vi "TLB Native Dynamic Events ver 0.08c.vi"() -> ()   [LabVIEW 2018]
uses:
  Labview Training Phase 2/Enum Controls/States for Action Engine.ctl
  Type def/TLB event states.ctl
  Type def/TLB MHL States.ctl
  <vilib>/Studica/Studica Toolkit/Background/I2C Channel.ctl
  <vilib>/myRIO/Common/Instrument Driver Framework/myRIO v1.0/AI/typedefs/AI Channels Enum.ctl
  <vilib>/myRIO/Common/Instrument Driver Framework/myRIO v1.0/AI/typedefs/AI Channels List.ctl
  Type def/Type def.ctl
  <vilib>/Studica/Studica Blackhawk/Blackhawk.lvlib
  <vilib>/Studica/Studica Toolkit/Background/Mxp Selection.ctl
  <vilib>/Studica/Studica Toolkit/Background/DIO Channel.ctl
  <vilib>/NI_Real-Time Target Support.lvlib
  <vilib>/ptbypt/NI_PtbyPt.lvlib
  <vilib>/addons/control/pid/NI_PID_pid.lvlib
  Underlying VI's/Webcam FGV Low level ver/State control.ctl
  <vilib>/userdefined/High Color/IMAQdx.ctl
  <vilib>/Studica/Studica Toolkit/NavX/NavX.lvlib
  <vilib>/addons/control/pid/pid.llb/PID (DBL).vi
panel:
  out "Displacement":T1
  out "Yaw":dbl
  out "Speed and distance cluster":T2
  out "Output":dbl
  in  "SENSOR":bool
  out "Decision":i8
  out "Manual Zero Yaw":bool
  in  "error in (no error)":errorcluster
  in  "RED LED State":enum16{"OFF", "ON", "BLINK"}(ring)
  in  "GREEN LED State":enum16{"OFF", "ON", "BLINK"}(ring)
  in  "Red LED":bool
  in  "Green LED":bool
  out "Input state":i8
  out "Waveform Chart 2":dbl(graph)
  out "Waveform Chart":dbl(graph)
  in  "STOP":bool
  out "DIO 0":bool
  out "DIO 1":bool
  out "Limit Switch Array":bool[](array[boolean])
  out "error out":errorcluster
  out "L/R average":fxp<+,64,64>
  out "Right Ultrasonic":fxp<+,64,16>
  out "Left Ultrasonic":fxp<+,64,16>
  out "Right IR Sensor":dbl
  out "Left IR Sensor":dbl
  out "Object detection count":T3
  out "Camera error":errorcluster
  in  "Servo Angle":u8(slide) scale=0.0..180.0
  in  "On/Off":bool
  out "Error":errorcluster
  out "element":T4
  out "Action Queue Items":i32
  out "State Logic Queue Items":i32
  out "Action Queues items":string[](array[string])=["Hardware reset", "Software reset", ""]
  out "State logic":T5=enum."Task 2"
  out "Action State":string
  # "TLB FRAMEWORK STATUS"
  # "Camera Status Loop"
  # "Test Programme written by Calvin Loke    Dated: 28 Aug 2019\nTest Programme revised by Dr Alex See   Dated 30 Aug 2019\n\nProgramme version:   TLB Native Dynamic Events ver 0.04b.vi"
  # "Problems now:\nYaw does not work when code is in last state mode\nSlow acceleration due to loop rate?"
  # "Motor Control Loop"
  # "NAVX Control Loop"
  # "Blackhawk status"
  # "Sensor data"
  # "System Health Status Update"
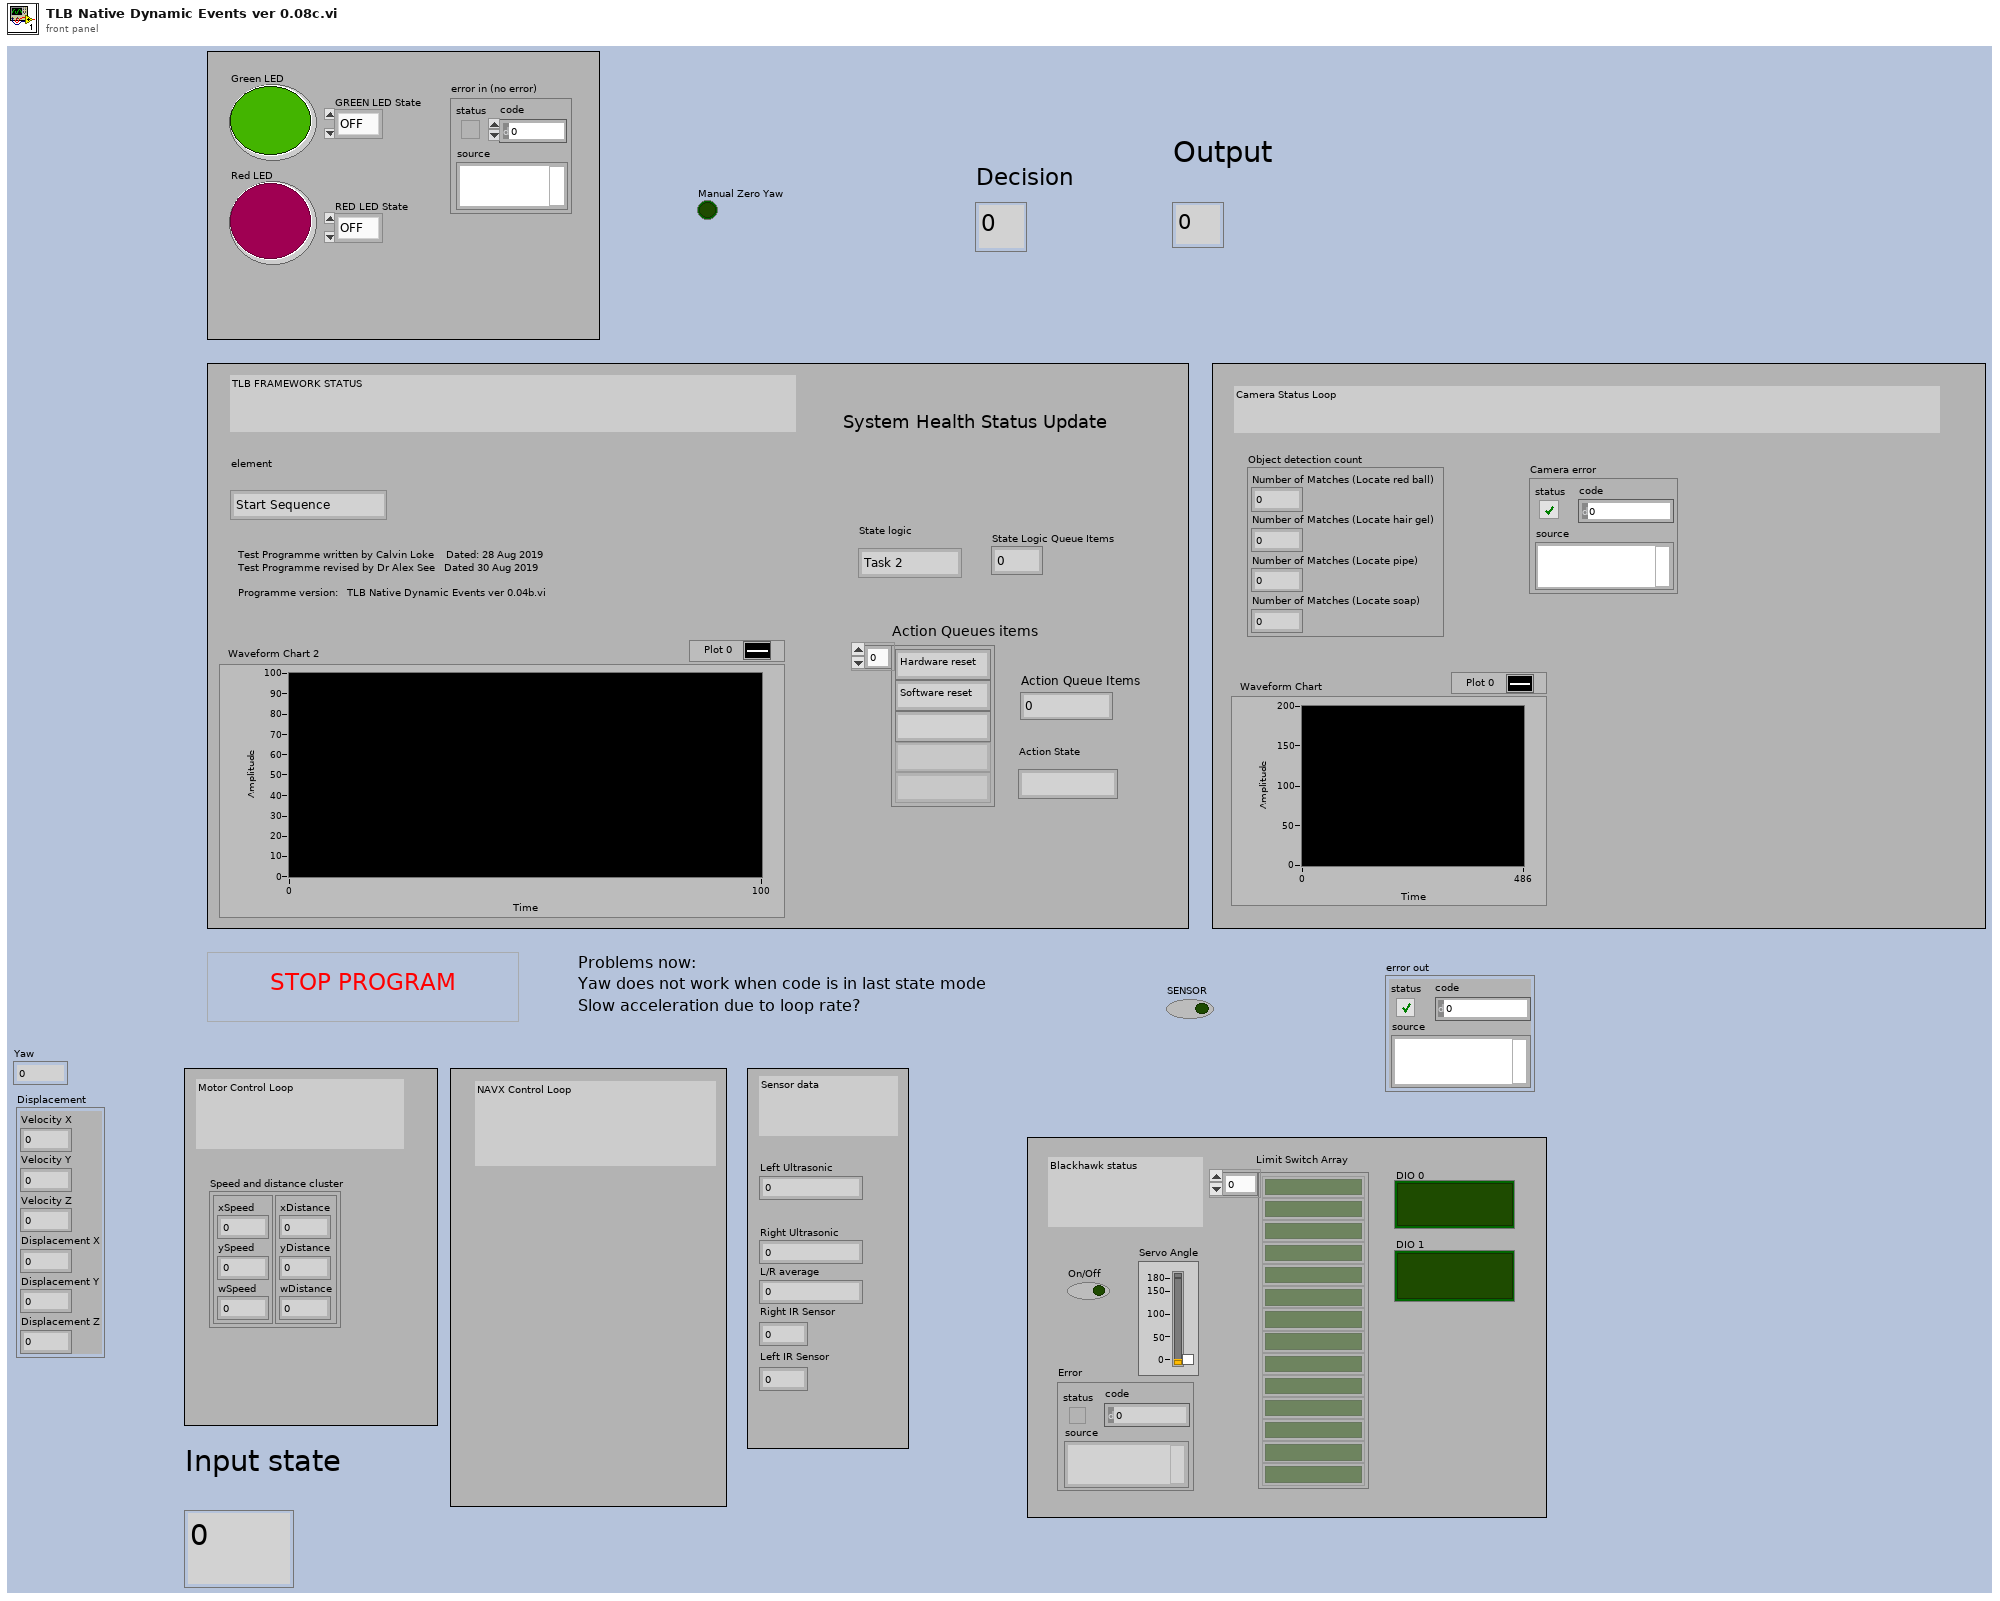
[diagram p1: front panel]
types:
  T1 = cluster{"Velocity X":dbl, "Velocity Y":dbl, "Velocity Z":dbl, "Displacement X":dbl, "Displacement Y":dbl, "Displacement Z":dbl}
  T2 = cluster{cluster{"xSpeed":dbl, "ySpeed":dbl, "wSpeed":dbl}, cluster{"xDistance":dbl, "yDistance":dbl, "wDistance":dbl}}
  T3 = cluster{"Number of Matches (Locate red ball)":i32, "Number of Matches (Locate hair gel)":i32, "Number of Matches (Locate pipe)":i32, "Number of Matches (Locate soap)":i32}
  T4 = typedef "TLB event states.ctl" = enum16{"Start Sequence", "Exit", "Start Task 1", "Start Task 2", "Start Task 3", "Start Task 4", "Camera vision", "Wall follow mode", "Idle", "Start Drive Straight"}
  T5 = typedef "TLB MHL States.ctl" = enum16{"None", "Startup", "Idle", "Processing", "Shutdown", "Reset", "Task 1", "Task 2", "Task 3", "Task 4", "Task 4a", "Task 4b", "Task 4c", "Task 4d", "Task 4e", "Task 4f", "Task 4g", "Task 4h", "Acquire image", "Wall follow mode", "Autodrive", "Autodrive a"}
  T6 = typedef "States for Action Engine.ctl" = enum16{"Initialize", "Write", "Read"}
  T7 = typedef "DIO Channel.ctl" = enum16{"Not Connected", "A/DIO1", "A/DIO2", "A/DIO3", "A/DIO4", "A/DIO5", "A/DIO6", "A/DIO7", "A/DIO13", "B/DIO1", "B/DIO2", "B/DIO3", "B/DIO4", "B/DIO5", "B/DIO6", "B/DIO7", "B/DIO13", "C/DIO0", "C/DIO1", "C/DIO2", "C/DIO3", "C/DIO4", "C/DIO5", "C/DIO6", "C/DIO7"}
  T8 = typedef "Type def.ctl" = cluster{"Front Ultrasonic Obstruct":bool, "Left Ultrasonic Obstruct":bool, "Right Ultrasonic Obstruct ":bool}
  T9 = typedef "I2C Channel.ctl" = enum16{"Not Connected", "A", "B"}
  T10 = enum16{"LAST STATE", "STOP", "FORWARD", "BACKWARD", "LEFT", "RIGHT", "RCW", "ACW", "INIT", "RESET ENCODERS"}
  T11 = cluster{"proportional gain (Kc)":dbl, "integral time (Ti, min)":dbl, "derivative time (Td, min)":dbl}
  T12 = typedef "State control.ctl" = enum16{"Initialise", "Start camera", "Continuous Acquisition ", "Stop camera", "Dispose all"}
  T13 = typedef "IMAQdx.ctl" = refnum<k21>
  T14 = typedef "Mxp Selection.ctl" = enum16{"MXP A", "MXP B"}
  T15 = enum16{"DISTANCE READ", "STOP", "FORWARD", "BACKWARD", "LEFT", "RIGHT", "RCW", "ACW", "INIT", "RESET ENCODERS"}
  T16 = typedef "AI Channels List.ctl" = T17[]
  T17 = typedef "AI Channels Enum.ctl" = enum16{"Not Connected", "AudioIn/Left", "AudioIn/Right", "C/AI0", "C/AI1", "A/AI0", "A/AI1", "A/AI2", "A/AI3", "A/AI4", "A/AI5", "A/AI6", "A/AI7", "B/AI0", "B/AI1", "B/AI2", "B/AI3", "B/AI4", "B/AI5", "B/AI6", "B/AI7", "AI/AI0", "AI/AI1", "AI/AI2", "AI/AI3", "A/AI0 (DIFF)", "A/AI1 (DIFF)", "A/AI2 (DIFF)", "A/AI3 (DIFF)", "B/AI0 (DIFF)", "B/AI1 (DIFF)", "B/AI2 (DIFF)", "B/AI3 (DIFF)"}
  T18 = cluster{"DIO Channel":T7, "FPGA VI Reference Out":refnum<k20>}
  T19 = typedef "Analog Scaling Constants List.ctl" = T20[]
  T20 = typedef "Analog Scaling Constants.ctl" = cluster{"LSB Weight (Volts)":dbl, "Offset (Volts)":dbl, "Signed?":bool}
  T21 = cluster{"Scale Constants Array":T19, "FPGA Reference Out":refnum<k20>, "AI Channel":T16}
  T22 = cluster{"I2C Channel":T9, "FPGA VI Reference Out":refnum<k20>}
  T23 = typedef "NI_Real-Time Target Support.lvlib/RT CPU Load.ctl" = cluster{"Total (%)":dbl, "Time Critical (%)":dbl, "Timed Structures (%)":dbl, "High (%)":dbl, "Above Normal (%)":dbl, "Normal (%)":dbl, "Background (%)":dbl, "Idle (%)":dbl, "ISR (%)":dbl}
  T24 = cluster{"CPU loads[0]":T23, "CPU loads[1]":T23, "CPU loads[2]":T23, "CPU loads[3]":T23, "CPU loads[4]":T23, "CPU loads[5]":T23, "CPU loads[6]":T23, "CPU loads[7]":T23, "CPU loads[8]":T23}
  T25 = cluster{"I2C Ref Out":cluster{"I2C Channel":T9, "FPGA VI Reference Out":refnum<k20>}, "Connected":bool, "Slave Address (7-bit)":u8, "Registry":u8[]}
  T26 = typedef "IMAQ Image.ctl" = refnum<image>
  T27 = cluster{"Yaw":dbl, "Roll":dbl, "Pitch":dbl, "Heading":dbl, "Fused Heading":dbl}
  T28 = cluster{"xDistance":dbl, "yDistance":dbl, "wDistance":dbl}
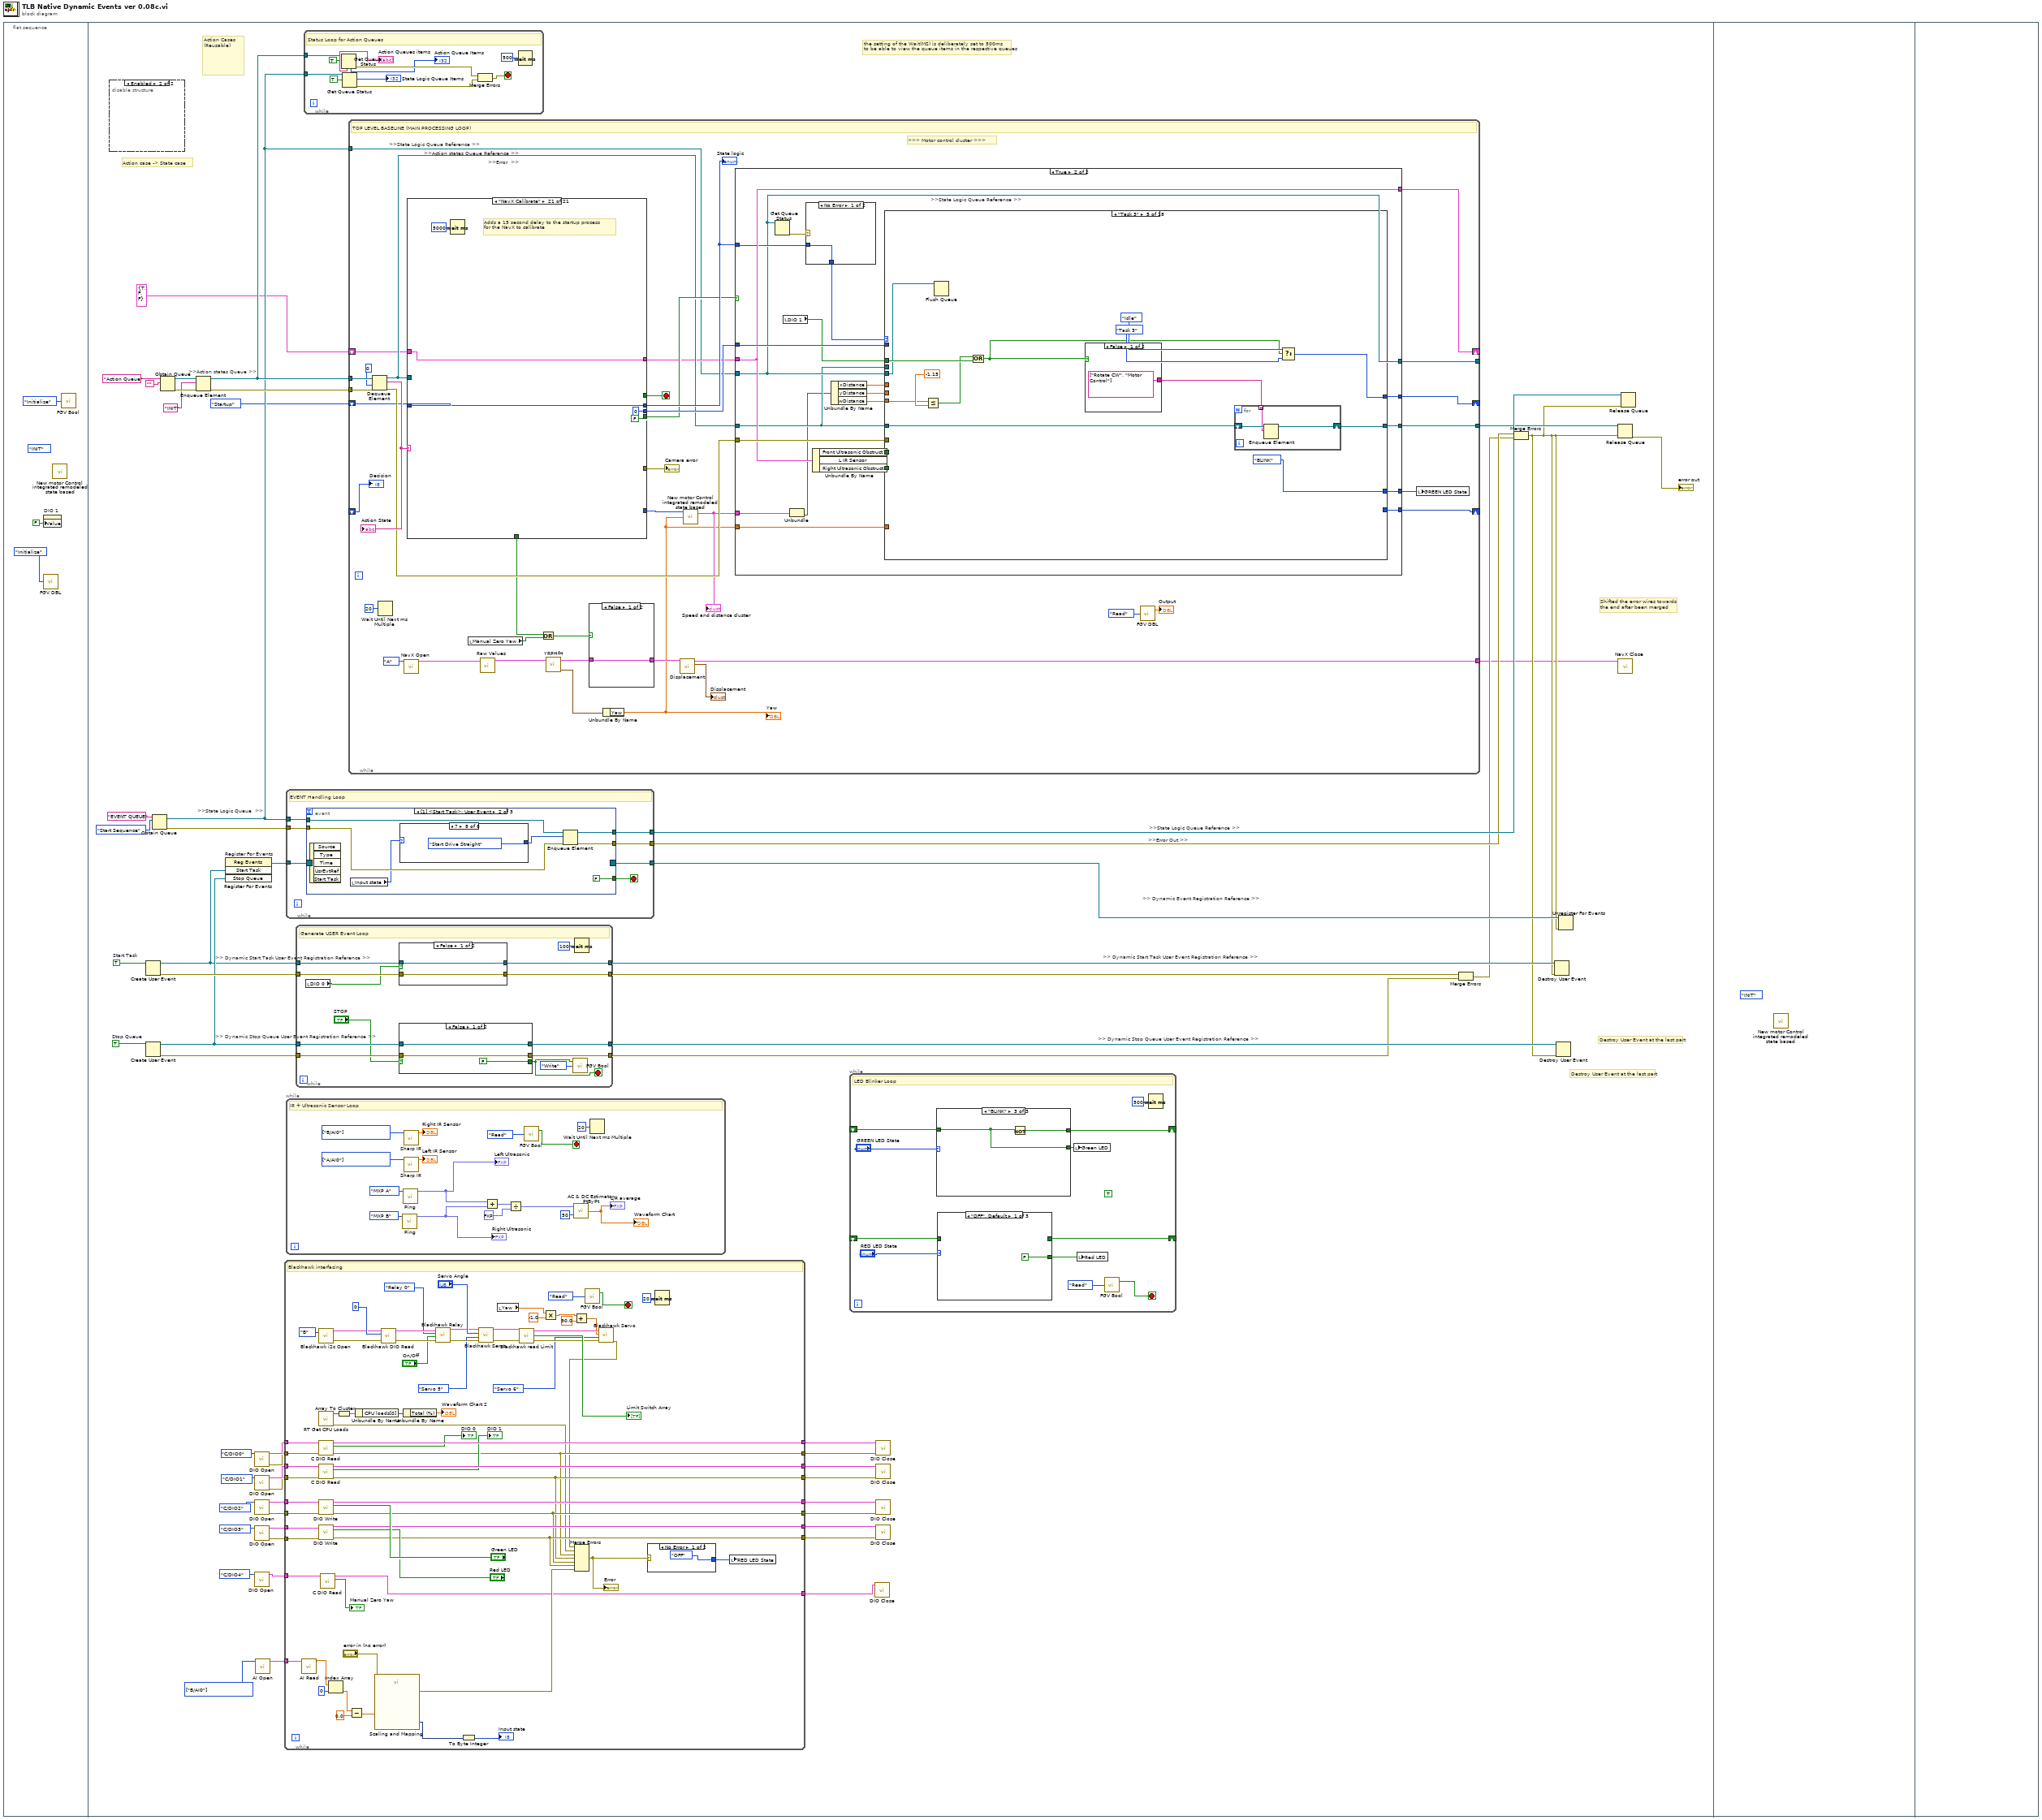
[diagram p0: block diagram]
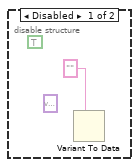
[diagram p2: hidden frame]
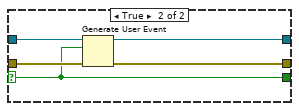
[diagram p3: hidden frame]
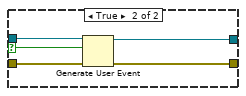
[diagram p4: hidden frame]
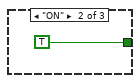
[diagram p5: hidden frame]
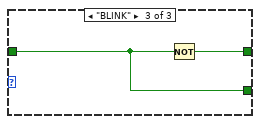
[diagram p6: hidden frame]
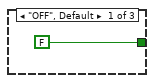
[diagram p7: hidden frame]
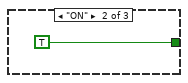
[diagram p8: hidden frame]
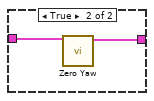
[diagram p9: hidden frame]
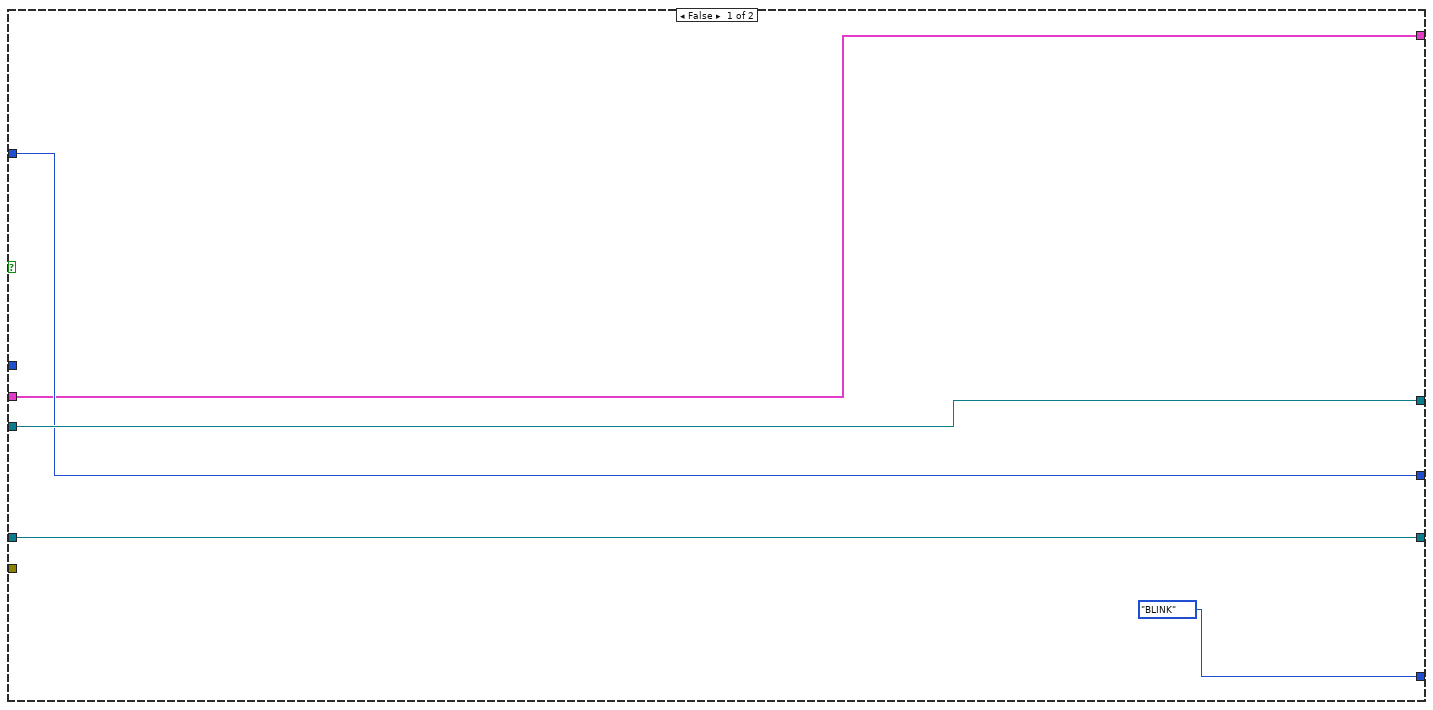
[diagram p10: hidden frame]
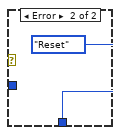
[diagram p11: hidden frame]
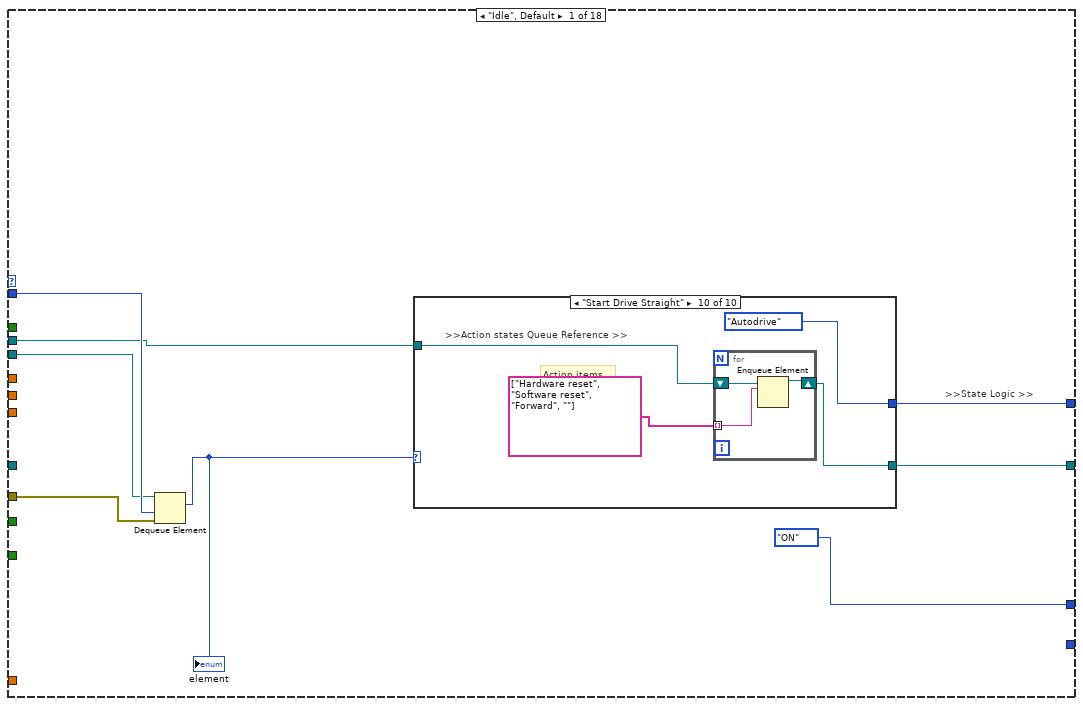
[diagram p12: hidden frame]
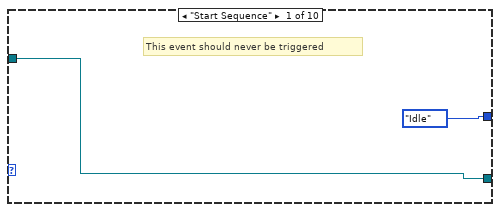
[diagram p13: hidden frame]
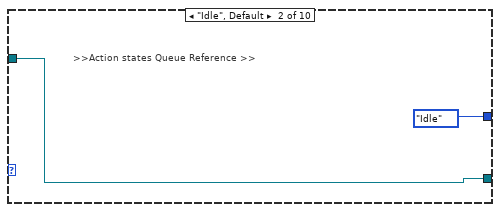
[diagram p14: hidden frame]
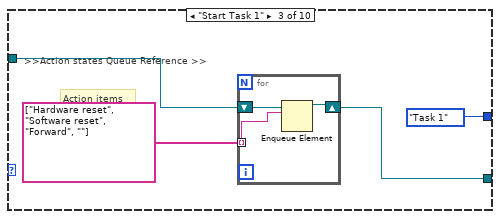
[diagram p15: hidden frame]
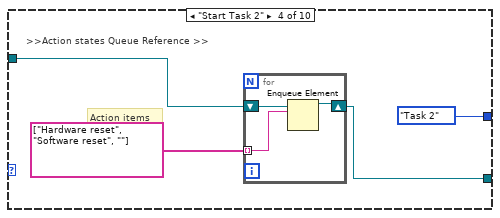
[diagram p16: hidden frame]
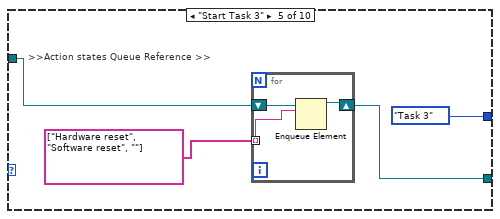
[diagram p17: hidden frame]
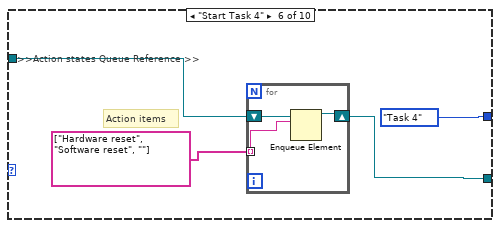
[diagram p18: hidden frame]
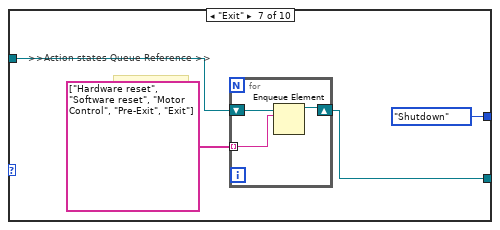
[diagram p19: hidden frame]
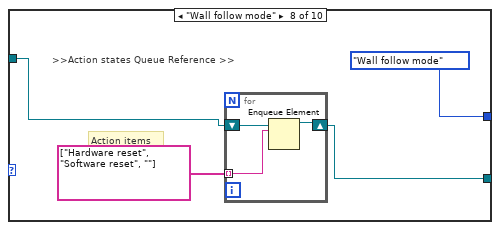
[diagram p20: hidden frame]
diagram:
  n1 = flat-sequence {
    frame #0 {
      (unwired) T15."INIT" ("States")
      n2 = call "FGV DBL.vi"("Init/Read/Write State"=States_for_Action_Engine."Initialize") -> ()  [unwired: 2 in, 2 out]
      n3 = property on="DIO 1" class="Bool (strict)"("Value"=FALSE ("DIO 1")) -> ()  [unwired: 2 in, 2 out]
      n4 = call "New motor Control integrated remodeled state based.vi"() -> ()  [unwired: 3 in, 2 out]
      n5 = call "FGV Bool.vi"("Init/Read/Write State"=States_for_Action_Engine."Initialize") -> ()  [unwired: 2 in, 2 out]
    }
    frame #1 {
      w13 = T16 [enum."B/AI0"] items=["Not Connected", "AudioIn/Left", "AudioIn/Right", "C/AI0", "C/AI1", "A/AI0", "A/AI1", "A/AI2", "A/AI3", "A/AI4", "A/AI5", "A/AI6", "A/AI7", "B/AI0", "B/AI1", "B/AI2", "B/AI3", "B/AI4", "B/AI5", "B/AI6", "B/AI7", "AI/AI0", "AI/AI1", "AI/AI2", "AI/AI3", "A/AI0 (DIFF)", "A/AI1 (DIFF)", "A/AI2 (DIFF)", "A/AI3 (DIFF)", "B/AI0 (DIFF)", "B/AI1 (DIFF)", "B/AI2 (DIFF)", "B/AI3 (DIFF)"] ("AI Channel")
      w60 = TRUE  # Stop Queue
      w59 = TRUE  # Start Task
      # "Action case -> State case"
      # "the setting of the Wait(MS) is deliberately set to 500ms\nto be able to view the queue items in the respective queues"
      # "Action Cases\n(Reusable)"
      # ">>Error Out >>"
      # ">> Dynamic Stop Queue User Event Registration Reference >>"
      # ">> Dynamic Start Task User Event Registration Reference >>"
      # ">> Dynamic Stop Queue User Event Registration Reference >>"
      # ">> Dynamic Start Task User Event Registration Reference >>"
      # ">> Dynamic Event Registration Reference >>"
      # ">>Action states Queue >>"
      # ">>State Logic Queue  >>"
      # ">>State Logic Queue Reference >>"
      # "Destroy User Event at the last part"
      # "Destroy User Event at the last part"
      # "Shifted the error wires towards\nthe end after been merged"
      n6 = disable-structure shown="Enabled" {
        frame Disabled {
          (unwired) variant
          (unwired) TRUE
          n7 = Variant To Data(type="") -> ()  [unwired: 2 in, 2 out]
        }
        frame Enabled {
        }
      }
      n8 = Create User Event(user event datatype=w59) -> (user event=w51:refnum<user-event>, error out=w56:errorcluster)  [unwired: 1 in]
      n9 = Create User Event(user event datatype=w60) -> (user event=w52:refnum<user-event>, error out=w55:errorcluster)  [unwired: 1 in]
      n10 = Obtain Queue(name (unnamed)="EVENT QUEUE", element data type=TLB_event_states."Start Sequence" ("Enum")) -> (queue out=w36:refnum<queue>, error out=w42:errorcluster)  [unwired: 3 in, 1 out]
      n11 = Obtain Queue(name (unnamed)="Action Queue", element data type="") -> (queue out=w45:refnum<queue>, error out=w41:errorcluster)  [unwired: 3 in, 1 out]
      n12 = Enqueue Element(queue=w45, element="INIT", error in (no error)=w41) -> (queue out=w37:refnum<queue>, error out=w40:errorcluster)  [unwired: 1 in, 1 out]
      n13 = register-events "Register For Events"(w51, w52) -> (reference out=w50:refnum<event-registration>)  [unwired: 2 in, 1 out]
      n14 = call <vilib>:"DIO Open.vi"("DIO Channel"=DIO_Channel."C/DIO4") -> ("DIO Info Out"=w7:T18)  [unwired: 9 in, 1 out]
      n15 = call <vilib>:"DIO Open.vi"("DIO Channel"=DIO_Channel."C/DIO0") -> ("error out"=w23:errorcluster, "DIO Info Out"=w29:T18)  [unwired: 9 in]
      n16 = call <vilib>:"DIO Open.vi"("DIO Channel"=DIO_Channel."C/DIO1") -> ("error out"=w21:errorcluster, "DIO Info Out"=w25:T18)  [unwired: 9 in]
      n17 = call <vilib>:"DIO Open.vi"("DIO Channel"=DIO_Channel."C/DIO2") -> ("error out"=w11:errorcluster, "DIO Info Out"=w17:T18)  [unwired: 9 in]
      n18 = call <vilib>:"DIO Open.vi"("DIO Channel"=DIO_Channel."C/DIO3") -> ("error out"=w9:errorcluster, "DIO Info Out"=w16:T18)  [unwired: 9 in]
      n19 = call <vilib>:"AI Open.vi"("AI Channel"=w13) -> ("Analog Info"=w12:T21)  [unwired: 9 in, 1 out]
      n20 = while {
        tunnel: w29 -> [w736]
        tunnel: [w735] -> w28
        tunnel: w25 -> [w734]
        tunnel: [w733] -> w24
        tunnel: w23 -> [w732]
        tunnel: [w701] -> w22
        tunnel: w21 -> [w731]
        tunnel: [w702] -> w20
        tunnel: w17 -> [w725]
        tunnel: w16 -> [w724]
        tunnel: [w721] -> w15
        tunnel: [w720] -> w14
        tunnel: w12 -> [w719]
        tunnel: w11 -> [w712]
        tunnel: [w703] -> w10
        tunnel: w9 -> [w711]
        tunnel: [w704] -> w8
        tunnel: w7 -> [w692]
        tunnel: [w691] -> w5
        stop <- w749 stop-if-true
        # "Blackhawk interfacing"
        n21 = call <vilib>:"AI Read.vi"("Analog Info"=w719) -> ("Array"=w715:dbl[])  [unwired: 9 in, 1 out]
        n22 = call <vilib>:"Blackhawk i2c Open.vi"("I2C Channel"=I2C_Channel."B") -> ("I2C Ref Out"=w727:T22, "error out"=w726:errorcluster)  [unwired: 2 in]
        n23 = call <vilib>:"RT Get CPU Loads.vi"() -> ("error out"=w700:errorcluster, "CPU loads"=w706:T23[])  [unwired: 10 in]
        n24 = call <vilib>:"C DIO Read.vi"("error in (no error)"=w732, "DIO Info In in"=w736) -> ("error out"=w701:errorcluster, "IN"=→"DIO 0":bool, "DIO Info In out"=w735:T18)  [unwired: 7 in]
        n25 = call <vilib>:"C DIO Read.vi"("error in (no error)"=w731, "DIO Info In in"=w734) -> ("error out"=w702:errorcluster, "IN"=→"DIO 1":bool, "DIO Info In out"=w733:T18)  [unwired: 7 in]
        n26 = call <vilib>:"DIO Write.vi"("error in (no error)"=w712, "Input"="Green LED", "DIO Info In"=w725) -> ("error out"=w703:errorcluster, "DIO Info Out"=w721:T18)  [unwired: 7 in]
        n27 = call <vilib>:"DIO Write.vi"("error in (no error)"=w711, "Input"="Red LED", "DIO Info In"=w724) -> ("error out"=w704:errorcluster, "DIO Info Out"=w720:T18)  [unwired: 7 in]
        n28 = call <vilib>:"C DIO Read.vi"("DIO Info In in"=w692) -> ("IN"=→"Manual Zero Yaw":bool, "DIO Info In out"=w691:T18)  [unwired: 8 in, 1 out]
        n29 = Index Array(array=w715, index=0) -> (element=w717:dbl)
        n30 = Array To Cluster(array=w706) -> (cluster=w707:T24)
        n31 = Subtract(x=w717, y=0.0) -> (x-y=w718:dbl)
        n32 = Unbundle By Name(w707) -> ("CPU loads[0]"=w708:T23)
        n33 = call "Scaling and Mapping"("error in (no error)"="error in (no error)", "Signals"=w718) -> ("error out"=w705:errorcluster, "Scaled Signals"=w713:dynamicdata)  [unwired: 8 in]
        n34 = call <vilib>:"Blackhawk DIO Read.vi"("I2C Ref In"=w727, "PIN"=u8 0, "error in (no error)"=w726) -> ("I2C Ref Out"=w747:T22, "error out"=w748:errorcluster)  [unwired: 3 in, 1 out]
        n35 = Unbundle By Name(w708) -> ("Total (%)"=→"Waveform Chart 2":dbl)
        n36 = call <vilib>:"Blackhawk Relay.vi"("error in (no error)"=w748, "On/Off"="On/Off", "Relay"=enum8{"Relay 0", "Relay 1", "Relay 2"}."Relay 0", "I2C Ref In"=w747) -> ("error out"=w744:errorcluster, "I2C Ref Out"=w741:T22)  [unwired: 6 in]
        n37 = To Byte Integer(number=w713) -> (8bit integer=→"Input state":i8)
        n38 = call <vilib>:"Blackhawk Servo.vi"("error in (no error)"=w744, "Servo Select"=enum16{"Servo 5", "Servo 6"}."Servo 5", "Servo Angle"="Servo Angle", "I2C Ref In"=w741) -> ("error out"=w739:errorcluster, "I2C Ref Out"=w738:T22)  [unwired: 6 in]
        n39 = local read "Yaw"() -> (w685:dbl)
        n40 = call <vilib>:"Blackhawk read Limit.vi"("error in (no error)"=w739, "I2C Ref In"=w738) -> ("error out"=w696:errorcluster, "Limit Switch Array"=→"Limit Switch Array":bool[], "I2C Ref Out"=w694:T22)  [unwired: 1 in]
        n41 = Multiply(x=w685, y=-1.0) -> (x*y=w687:dbl)
        n42 = Add(x=w687, y=90.0) -> (x+y=w688:dbl)
        n43 = call "FGV Bool.vi"("Init/Read/Write State"=States_for_Action_Engine."Read") -> ("Output node"=w749:bool)  [unwired: 2 in, 1 out]
        n44 = call <vilib>:"Blackhawk Servo.vi"("error in (no error)"=w696, "Servo Select"=enum16{"Servo 5", "Servo 6"}."Servo 6", "Servo Angle"=w688, "I2C Ref In"=w694) -> ("error out"=w695:errorcluster)  [unwired: 6 in, 1 out]
        n45 = Merge Errors(w695, w700, w701, w702, w703, w704, w705) -> (w699:errorcluster)
        "Error" <- w699
        n46 = case shown="No Error" w699 {
          tunnel: [enum16{"OFF", "ON", "BLINK"}."OFF" ("RED LED State") enum16{"OFF", "ON", "BLINK"}."BLINK" ("RED LED State")] -> w710
          frame No Error {
          }
          frame Error {
          }
        }
        n47 = Wait (ms)(milliseconds to wait=u32 20) -> ()  [unwired: 1 out]
        n48 = local write "RED LED State"(w710) -> ()
      }
      n49 = while {
        tunnel: w50 -> [w657]
        tunnel: [w656] -> w49
        tunnel: w36 -> [w654]
        tunnel: [w653] -> w48
        tunnel: w42 -> [w652]
        tunnel: [w651] -> w39
        stop <- w655 stop-if-true
        # "EVENT Handling Loop"
        n50 = event shown="[1] <Start Task>: User Event" {
          selector: w657 -> [_ _ _]
          dyn-events: [_ _ _] -> w656
          timeout: _ -> [_ _ _]
          tunnel: [FALSE FALSE w684] -> w655
          tunnel: w654 -> [w662 w669 w682]
          tunnel: [w661 w668 w683] -> w653
          tunnel: w652 -> [w659 w667 w680]
          tunnel: [w658 w666 w679] -> w651
          event Timeout {
            n51 = event-data() -> ()  [unwired: 1 in, 3 out]
            n52 = Enqueue Element(queue=w662, element=TLB_event_states."Idle" ("Enum"), error in (no error)=w659) -> (queue out=w661:refnum<queue>, error out=w658:errorcluster)  [unwired: 1 in, 1 out]
          }
          event User Event {
            n53 = event-data() -> ()  [unwired: 1 in, 5 out]
            n54 = local read "Input state"() -> (w665:i8)
            n55 = case shown="7" w665 {
              tunnel: [TLB_event_states."Idle" ("Enum") TLB_event_states."Start Task 1" ("Enum") TLB_event_states."Start Task 2" ("Enum") TLB_event_states."Start Task 3" ("Enum") TLB_event_states."Start Task 4" ("Enum") TLB_event_states."Wall follow mode" ("Enum") TLB_event_states."Camera vision" ("Enum") TLB_event_states."Start Drive Straight" ("Enum")] -> w664
              frame 0 {
              }
              frame 1 {
              }
              frame 2 {
              }
              frame 3, Default {
              }
              frame 4 {
              }
              frame 5 {
              }
              frame 6 {
              }
              frame 7 {
              }
            }
            n56 = Enqueue Element(queue=w669, element=w664, error in (no error)=w667) -> (queue out=w668:refnum<queue>, error out=w666:errorcluster)  [unwired: 1 in, 1 out]
          }
          event User Event {
            n57 = event-data() -> ("Stop Queue"=w684:bool)  [unwired: 1 in, 4 out]
            n58 = Enqueue Element At Opposite End(queue=w682, element=TLB_event_states."Exit" ("Enum"), error in (no error)=w680) -> (queue out=w683:refnum<queue>, error out=w679:errorcluster)  [unwired: 1 in, 1 out]
          }
        }
      }
      n59 = while {
        stop <- w644 stop-if-true
        w649 = T16 [enum."A/AI0"] items=["Not Connected", "AudioIn/Left", "AudioIn/Right", "C/AI0", "C/AI1", "A/AI0", "A/AI1", "A/AI2", "A/AI3", "A/AI4", "A/AI5", "A/AI6", "A/AI7", "B/AI0", "B/AI1", "B/AI2", "B/AI3", "B/AI4", "B/AI5", "B/AI6", "B/AI7", "AI/AI0", "AI/AI1", "AI/AI2", "AI/AI3", "A/AI0 (DIFF)", "A/AI1 (DIFF)", "A/AI2 (DIFF)", "A/AI3 (DIFF)", "B/AI0 (DIFF)", "B/AI1 (DIFF)", "B/AI2 (DIFF)", "B/AI3 (DIFF)"] ("AI Channel")
        w650 = T16 [enum."B/AI0"] items=["Not Connected", "AudioIn/Left", "AudioIn/Right", "C/AI0", "C/AI1", "A/AI0", "A/AI1", "A/AI2", "A/AI3", "A/AI4", "A/AI5", "A/AI6", "A/AI7", "B/AI0", "B/AI1", "B/AI2", "B/AI3", "B/AI4", "B/AI5", "B/AI6", "B/AI7", "AI/AI0", "AI/AI1", "AI/AI2", "AI/AI3", "A/AI0 (DIFF)", "A/AI1 (DIFF)", "A/AI2 (DIFF)", "A/AI3 (DIFF)", "B/AI0 (DIFF)", "B/AI1 (DIFF)", "B/AI2 (DIFF)", "B/AI3 (DIFF)"] ("AI Channel")
        # "IR + Ultrasonic Sensor Loop"
        n60 = call <vilib>:"Ping.vi"("Mxp Side"=Mxp_Selection."MXP B") -> ("CM"=w638:fxp<+,64,16>)  [unwired: 8 in, 2 out]
        "Right Ultrasonic" <- w638
        n61 = call <vilib>:"Ping.vi"("Mxp Side"=Mxp_Selection."MXP A") -> ("CM"=w639:fxp<+,64,16>)  [unwired: 8 in, 2 out]
        "Left Ultrasonic" <- w639
        n62 = call <vilib>:"Sharp IR.vi"("AI Channel"=w650) -> ("Sharp IR Distance"=→"Right IR Sensor":dbl)  [unwired: 8 in, 2 out]
        n63 = call <vilib>:"Sharp IR.vi"("AI Channel"=w649) -> ("Sharp IR Distance"=→"Left IR Sensor":dbl)  [unwired: 8 in, 2 out]
        n64 = Add(x=w639, y=w638) -> (x+y=w641:fxp<+,64,17>)
        n65 = Divide(x=w641, y=fxp<+,64,17> 2.0) -> (x/y=w637:fxp<+,64,64>)
        n66 = call "FGV Bool.vi"("Init/Read/Write State"=States_for_Action_Engine."Read") -> ("Output node"=w644:bool)  [unwired: 2 in, 1 out]
        n67 = call <vilib>:"AC & DC Estimator PtByPt.vi"("signal"=w637, "sample length"=50) -> ("DC estimate (V)"=→"L/R average" →"Waveform Chart":dbl)  [unwired: 1 in, 2 out]
        n68 = Wait Until Next ms Multiple(millisecond multiple=u32 20) -> ()  [unwired: 1 out]
      }
      n69 = while {
        tunnel: w51 -> [w84]
        tunnel: w52 -> [w83]
        tunnel: [w82] -> w58
        tunnel: [w81] -> w57
        tunnel: w56 -> [w80]
        tunnel: [w79] -> w54
        tunnel: w55 -> [w78]
        tunnel: [w77] -> w53
        stop <- w75 stop-if-true
        # "Generate USER Event Loop"
        n70 = local read "DIO 0"() -> (w74:bool)
        n71 = case shown="False" w74 {
          selector: w74 -> [_ w96]
          tunnel: w84 -> [w95 w100]
          tunnel: [w95 w99] -> w81
          tunnel: w80 -> [w94 w98]
          tunnel: [w94 w97] -> w79
          frame False {
          }
          frame True {
            n72 = Generate User Event(user event=w100, event data cluster=w96, error in=w98) -> (user event out=w99:refnum<user-event>, error out=w97:errorcluster)  [unwired: 1 in]
          }
        }
        n73 = case shown="False" "STOP" {
          selector: "STOP" -> [_ w89]
          tunnel: w83 -> [w88 w93]
          tunnel: [w88 w92] -> w82
          tunnel: w78 -> [w87 w91]
          tunnel: [w87 w90] -> w77
          tunnel: [FALSE w89] -> w75
          frame False {
          }
          frame True {
            n74 = Generate User Event(user event=w93, event data cluster=w89, error in=w91) -> (user event out=w92:refnum<user-event>, error out=w90:errorcluster)  [unwired: 1 in]
          }
        }
        n75 = call "FGV Bool.vi"("Init/Read/Write State"=States_for_Action_Engine."Write", "Input Node"=w75) -> ()  [unwired: 1 in, 2 out]
        n76 = Wait (ms)(milliseconds to wait=u32 100) -> ()  [unwired: 1 out]
      }
      n77 = while {
        tunnel: w37 -> [w70]
        tunnel: w36 -> [w67]
        stop <- w64 stop-if-true
        # "Status Loop for Action Queues"
        n78 = Get Queue Status(queue=w70, return elements? (F)=TRUE) -> (error out=w66:errorcluster, # elements in queue=→"Action Queue Items":i32, elements=→"Action Queues items":string[])  [unwired: 1 in, 5 out]
        n79 = Get Queue Status(queue=w67, return elements? (F)=TRUE) -> (# pending remove=→"State Logic Queue Items":i32, error out=w65:errorcluster)  [unwired: 1 in, 6 out]
        n80 = Merge Errors(w66, w65) -> (w64:errorcluster)
        n81 = Wait (ms)(milliseconds to wait=u32 500) -> ()  [unwired: 1 out]
      }
      n82 = while {
        tunnel: w36 -> [w141]
        shift-right: [w152] -> _
        shift-left: TLB_MHL_States."Startup" ("Enum") -> [w146]
        tunnel: w37 -> [w157]
        tunnel: w40 -> [w155]
        tunnel: [w154] -> _
        tunnel: [w153] -> w32
        shift-right: [w143] -> _
        shift-left: T8 {"Front Ultrasonic Obstruct"=TRUE, "Left Ultrasonic Obstruct"=FALSE, "Right Ultrasonic Obstruct "=FALSE} -> [w145]
        shift-right: [w135] -> _
        shift-left: _ -> [w134]
        tunnel: [w123] -> w4
        stop <- w139 stop-if-true
        # ">>> Motor control cluster >>>"
        # ">>Error  >>"
        # ">>Action states Queue Reference >>"
        # ">>State Logic Queue Reference >>"
        # "TOP LEVEL BASELINE (MAIN PROCESSING LOOP)"
        n83 = Dequeue Element(queue=w157, timeout in ms (-1)=0, error in (no error)=w155) -> (queue out=w147:refnum<queue>, element=w156:string, error out=w148:errorcluster)  [unwired: 1 out]
        "Action State" <- w156
        n84 = Wait Until Next ms Multiple(millisecond multiple=u32 20) -> ()  [unwired: 1 out]
        n85 = call <vilib>:"NavX Open.vi"("I2C Channel"=I2C_Channel."A") -> ("NavX Info"=w127:T25)  [unwired: 9 in, 1 out]
        n86 = case shown="\"NavX Calibrate\"" w156 {
          tunnel: [w489 w504 w510 w515 w520 w526 w531 w534 w541 w546 w556 w563 TLB_MHL_States."Shutdown" ("Enum") w573 w584 w587 w598 w609 w617 w629 w633] -> w158
          tunnel: [w492 0 0 0 0 0 0 0 0 0 0 0 0 0 0 0 0 0 0 0 0] -> w151
          tunnel: [TRUE FALSE FALSE FALSE FALSE FALSE FALSE FALSE FALSE FALSE FALSE FALSE FALSE FALSE FALSE FALSE FALSE FALSE FALSE FALSE FALSE] -> w150
          tunnel: w147 -> [_ _ _ _ _ _ _ _ _ _ _ _ _ _ _ _ _ _ _ _ _]
          tunnel: w146 -> [w489 w504 w510 w515 w520 w526 w531 w534 w541 w546 w556 w563 _ w573 w584 w587 w598 w609 w617 w629 w633]
          tunnel: w145 -> [w490 w499 w507 w516 w518 w523 w528 w533 w538 w544 w553 w560 w566 w574 w583 w590 w599 w610 w616 w626 w634]
          tunnel: [w490 w498 w506 w516 w518 w523 w528 w533 w538 w544 w552 w560 w566 w574 w580 w589 w599 w610 w616 w626 w634] -> w144
          tunnel: [_ _ _ _ _ _ _ _ _ _ _ _ _ _ _ _ _ w600 w612 w620 _] -> w142
          tunnel: [_ _ _ _ _ _ _ _ _ _ _ _ TRUE _ _ _ _ _ _ _ _] -> w139
          tunnel: [T10."LAST STATE" ("Move mode") T10."INIT" ("Move mode") T10."FORWARD" ("Move mode") T10."LAST STATE" ("Move mode") T10."BACKWARD" ("Move mode") T10."RIGHT" ("Move mode") T10."LEFT" ("Move mode") T10."RCW" ("Move mode") T10."ACW" ("Move mode") T10."STOP" ("Move mode") _ T10."RESET ENCODERS" ("Move mode") T10."INIT" ("Move mode") T10."INIT" ("Move mode") _ _ _ _ _ _ _] -> w137
          tunnel: [FALSE ("NavX Zero Yaw") _ _ _ _ _ _ _ _ FALSE ("NavX Zero Yaw") FALSE ("NavX Zero Yaw") TRUE ("NavX Zero Yaw") _ _ _ _ _ _ _ _ _] -> w120
          frame "No action", Default {
            n87 = case shown="\"Startup\", Default" w489 {
              tunnel: [0 100] -> w492
              frame "Startup", Default {
              }
              frame "Idle" {
              }
            }
          }
          frame "Init" {
            # ">>State Logic  >>"
            n88 = local write "Servo Angle"(u8 90 ("Servo Angle")) -> ()
            n89 = Bundle By Name(cluster=w499, "Front Ultrasonic Obstruct"=FALSE ("Object detected"), "L IR Sensor"=0.0, "Right Ultrasonic Obstruct"=FALSE ("In move state?")) -> (w498:T8)
          }
          frame "Forward" {
            n90 = Bundle By Name(cluster=w507, "Right Ultrasonic Obstruct"=TRUE ("In move state?")) -> (w506:T8)
          }
          frame " Motor Control" {
          }
          frame "Reverse" {
          }
          frame "Right" {
          }
          frame "Left" {
          }
          frame "Rotate CW" {
          }
          frame "Rotate ACW" {
          }
          frame "Stop" {
          }
          frame "Software reset" {
            w548 = FALSE ("In move state?")
            # "Resets any software variables\nand/or non-critical states"
            n91 = Wait (ms)(milliseconds to wait=u32 20) -> ()  [unwired: 1 out]
            n92 = Bundle By Name(cluster=w553, "Front Ultrasonic Obstruct"=w548, "L IR Sensor"=0.0, "Right Ultrasonic Obstruct"=w548) -> (w552:T8)
          }
          frame "Hardware reset" {
            n93 = Wait (ms)(milliseconds to wait=u32 100) -> ()  [unwired: 1 out]
          }
          frame "Exit" {
          }
          frame "Pre-Exit" {
          }
          frame "Ultrasonic read" {
            # "Object detection"
            n94 = local read "L/R average"() -> (w578:fxp<+,64,64>)
            n95 = Less Or Equal?(x=w578, y=35.0) -> (x <= y?=w577:bool)
            n96 = Or(x=w577, y="SENSOR") -> (x .or. y?=w576:bool)
            n97 = Bundle By Name(cluster=w583, "Front Ultrasonic Obstruct"=w576) -> (w580:T8)
          }
          frame "IR Sensor Read" {
            n98 = local read "Left IR Sensor"() -> (w588:dbl)
            n99 = Bundle By Name(cluster=w590, "L IR Sensor"=w588) -> (w589:T8)
          }
          frame "Calculate" {
            n100 = Unbundle By Name(w599) -> ("L IR Sensor"=w594:dbl)
            n101 = call-poly <vilib>:"PID.vi"("output range"=cluster{"output high":dbl, "output low":dbl} {"output high"=0.3, "output low"=-0.3}, "PID gains"=T11 {"proportional gain (Kc)"=0.01, "integral time (Ti, min)"=0.0, "derivative time (Td, min)"=0.0}, "process variable"=w594, "setpoint"=20.0) -> ("output"=w591:dbl)  [unwired: 6 in, 1 out]
            n102 = Negate(x=w591) -> ()  [unwired: 1 out]
          }
          frame "Cam Init" {
            n103 = call "Low-Level Grab.vi"("States"=State_control."Initialise", "Session In"=T13 "cam1") -> ("error out"=w601:errorcluster, "Session Out"=w602:T13)  [unwired: 7 in, 1 out]
            n104 = call "Low-Level Grab.vi"("error in (no error)"=w601, "States"=State_control."Start camera", "Session In"=w602) -> ("error out"=w600:errorcluster)  [unwired: 6 in, 2 out]
            n105 = local write "Servo Angle"(u8 170 ("Servo Angle")) -> ()
          }
          frame "Cam Acq" {
            n106 = call "Low-Level Grab.vi"("States"=State_control."Continuous Acquisition ") -> ("error out"=w613:errorcluster, "Image Out"=w614:T26)  [unwired: 8 in, 1 out]
            n107 = call "All object detection ver2.vi"("Image In"=w614, "error in"=w613) -> ("Object detection count"=→"Object detection count":T3, "error out"=w612:errorcluster)  [unwired: 1 out]
          }
          frame "Cam Exit" {
            n108 = call "Low-Level Grab.vi"("States"=State_control."Stop camera") -> ("error out"=w621:errorcluster, "Session Out"=w623:T13)  [unwired: 8 in, 1 out]
            n109 = local write "Servo Angle"(u8 90 ("Servo Angle")) -> ()
            n110 = call "Low-Level Grab.vi"("error in (no error)"=w621, "States"=State_control."Dispose all", "Session In"=w623) -> ("error out"=w620:errorcluster)  [unwired: 6 in, 2 out]
          }
          frame "NavX Calibrate" {
            # "Adds a 15 second delay to the startup process \nfor the NavX to calibrate"
            n111 = Wait (ms)(milliseconds to wait=u32 5000) -> ()  [unwired: 1 out]
          }
        }
        "State logic" <- w158
        "Camera error" <- w142
        n112 = local read "Manual Zero Yaw"() -> (w121:bool)
        n113 = call <vilib>:"Raw Values.vi"("NavX Info In"=w127) -> ("NavX Info Out"=w130:T25)  [unwired: 8 in, 1 out]
        n114 = Or(x=w120, y=w121) -> (x .or. y?=w122:bool)
        n115 = call <vilib>:"YRPHfH.vi"("NavX Info In"=w130) -> ("YRPHfH"=w131:T27, "NavX Info Out"=w129:T25)  [unwired: 3 in]
        n116 = case shown="False" w122 {
          tunnel: [w159 w161] -> w126
          tunnel: w129 -> [w159 w160]
          frame False {
          }
          frame True {
            n117 = call <vilib>:"Zero Yaw.vi"("NavX Info In"=w160) -> ("NavX Info Out"=w161:T25)  [unwired: 10 in]
          }
        }
        n118 = Unbundle By Name(w131) -> ("Yaw"=w124:dbl)
        "Yaw" <- w124
        n119 = call <vilib>:"Displacement.vi"("NavX Info In"=w126) -> ("Displacement"=→"Displacement":T1, "NavX Info Out"=w123:T25)  [unwired: 9 in]
        n120 = call "New motor Control integrated remodeled state based.vi"("Yaw"=w124, "States"=w137) -> ("Speed and distance cluster"=w136:T2)  [unwired: 1 in, 1 out]
        "Speed and distance cluster" <- w136
        n121 = case shown="True" w150 {
          tunnel: w158 -> [w165 w177]
          tunnel: w141 -> [w166 w176]
          tunnel: w147 -> [w164 w172]
          tunnel: [w166 w176] -> w154
          tunnel: [w164 w187] -> w153
          tunnel: [w165 w186] -> w152
          tunnel: w148 -> [_ w185]
          tunnel: w151 -> [_ w184]
          tunnel: w144 -> [w163 w179]
          tunnel: [w163 w179] -> w143
          tunnel: [enum16{"OFF", "ON", "BLINK"}."BLINK" ("GREEN LED State") w173] -> w138
          tunnel: w136 -> [_ w170]
          tunnel: [_ w168] -> w135
          tunnel: w124 -> [_ w167]
          frame False {
          }
          frame True {
            # ">>State Logic Queue Reference >>"
            n122 = Get Queue Status(queue=w176) -> (error out=w175:errorcluster)  [unwired: 2 in, 7 out]
            n123 = local read "DIO 1"() -> (w174:bool)
            n124 = Unbundle(w170) -> (w169:T28)  [unwired: 1 out]
            n125 = case shown="No Error" w175 {
              tunnel: [w188 TLB_MHL_States."Reset" ("Enum")] -> w178
              tunnel: w177 -> [w188 _]
              frame No Error {
              }
              frame Error {
              }
            }
            n126 = Unbundle By Name(w179) -> ("Front Ultrasonic Obstruct"=w180:bool, "Right Ultrasonic Obstruct"=w171:bool)  [unwired: 1 out]
            n127 = Unbundle By Name(w169) -> ("xDistance"=w181:dbl, "yDistance"=w183:dbl, "wDistance"=w182:dbl)
            n128 = case shown="\"Task 3\"" w178 {
              tunnel: w176 -> [w193 w258 w269 w286 w305 w321 w336 w352 w368 w384 _ w408 w430 w443 _ _ _ _]
              tunnel: w172 -> [_ w261 w275 w290 w314 w325 w341 w358 w373 w390 w401 w411 w431 w447 w456 w460 w466 w480]
              tunnel: [w190 w260 w274 w291 w313 w326 w340 w357 w372 w389 w400 w412 w432 w446 w456 w459 w466 w481] -> w187
              tunnel: [w196 TLB_MHL_States."Idle" ("Enum") w277 w292 w310 w329 w343 w356 w374 w388 TLB_MHL_States."Shutdown" ("Enum") w414 w423 w445 TLB_MHL_States."Reset" ("Enum") TLB_MHL_States."Shutdown" ("Enum") TLB_MHL_States."Reset" ("Enum") w477] -> w186
              tunnel: w185 -> [w194 _ _ _ _ _ _ _ _ _ _ _ _ _ _ _ _ _]
              tunnel: w184 -> [w195 _ _ _ _ _ _ _ _ _ _ _ _ _ _ _ _ _]
              tunnel: w174 -> [_ _ w272 w289 w308 _ _ _ _ w387 _ w409 w426 w444 _ _ _ w469]
              tunnel: w183 -> [_ _ w267 _ _ _ w335 w351 _ _ _ _ _ _ _ _ _ _]
              tunnel: w182 -> [_ _ _ _ w303 _ _ _ _ _ _ _ _ _ _ _ _ _]
              tunnel: w181 -> [_ _ _ _ _ _ _ _ w367 _ _ _ _ _ _ _ _ _]
              tunnel: w180 -> [_ _ _ w287 _ w323 _ _ _ w386 _ _ w425 _ _ _ _ _]
              tunnel: [enum16{"OFF", "ON", "BLINK"}."ON" ("GREEN LED State") enum16{"OFF", "ON", "BLINK"}."OFF" ("GREEN LED State") enum16{"OFF", "ON", "BLINK"}."BLINK" ("GREEN LED State") enum16{"OFF", "ON", "BLINK"}."BLINK" ("GREEN LED State") enum16{"OFF", "ON", "BLINK"}."BLINK" ("GREEN LED State") enum16{"OFF", "ON", "BLINK"}."BLINK" ("GREEN LED State") enum16{"OFF", "ON", "BLINK"}."BLINK" ("GREEN LED State") enum16{"OFF", "ON", "BLINK"}."BLINK" ("GREEN LED State") enum16{"OFF", "ON", "BLINK"}."BLINK" ("GREEN LED State") enum16{"OFF", "ON", "BLINK"}."BLINK" ("GREEN LED State") enum16{"OFF", "ON", "BLINK"}."OFF" ("GREEN LED State") enum16{"OFF", "ON", "BLINK"}."BLINK" ("GREEN LED State") enum16{"OFF", "ON", "BLINK"}."BLINK" ("GREEN LED State") enum16{"OFF", "ON", "BLINK"}."BLINK" ("GREEN LED State") _ enum16{"OFF", "ON", "BLINK"}."OFF" ("GREEN LED State") _ _] -> w173
              tunnel: w172 -> [w191 _ _ _ _ _ _ _ _ _ _ _ _ _ _ _ _ _]
              tunnel: w171 -> [_ _ _ _ _ _ _ _ _ _ _ _ _ _ _ _ _ _]
              tunnel: [_ _ _ _ _ _ _ _ _ _ _ _ w421 _ _ _ _ _] -> w168
              tunnel: w167 -> [_ _ _ _ _ _ _ _ _ _ _ _ _ _ _ _ _ w468]
              frame "Idle", Default {
                # ">>State Logic >>"
                n129 = Dequeue Element(queue=w193, timeout in ms (-1)=w195, error in (no error)=w194) -> (element=w197:T4)  [unwired: 3 out]
                "element" <- w197
                n130 = case shown="\"Start Drive Straight\"" w197 {
                  tunnel: [TLB_MHL_States."Idle" ("Enum") TLB_MHL_States."Idle" ("Enum") TLB_MHL_States."Task 1" ("Enum") TLB_MHL_States."Task 2" ("Enum") TLB_MHL_States."Task 3" ("Enum") TLB_MHL_States."Task 4" ("Enum") TLB_MHL_States."Shutdown" ("Enum") TLB_MHL_States."Wall follow mode" ("Enum") TLB_MHL_States."Acquire image" ("Enum") TLB_MHL_States."Autodrive" ("Enum")] -> w196
                  tunnel: w191 -> [w198 w200 w204 w211 w217 w225 w232 w239 w246 w253]
                  tunnel: [w198 w200 w203 w210 w218 w224 w231 w238 w245 w251] -> w190
                  frame "Start Sequence" {
                    # "This event should never be triggered"
                  }
                  frame "Idle", Default {
                    # ">>Action states Queue Reference >>"
                  }
                  frame "Start Task 1" {
                    # ">>Action states Queue Reference >>"
                    # "Action items"
                    n131 = for {
                      shift-right: [w208] -> w203
                      shift-left: w204 -> [w207]
                      tunnel: string[] ["Hardware reset", "Software reset", "Forward", ""] -> [w206] mode=indexing
                      n132 = Enqueue Element(queue=w207, element=w206) -> (queue out=w208:refnum<queue>)  [unwired: 2 in, 2 out]
                    }
                  }
                  frame "Start Task 2" {
                    # ">>Action states Queue Reference >>"
                    # "Action items"
                    n133 = for {
                      shift-right: [w215] -> w210
                      shift-left: w211 -> [w214]
                      tunnel: string[] ["Hardware reset", "Software reset", ""] -> [w213] mode=indexing
                      n134 = Enqueue Element(queue=w214, element=w213) -> (queue out=w215:refnum<queue>)  [unwired: 2 in, 2 out]
                    }
                  }
                  frame "Start Task 3" {
                    # ">>Action states Queue Reference >>"
                    n135 = for {
                      shift-right: [w222] -> w218
                      shift-left: w217 -> [w221]
                      tunnel: string[] ["Hardware reset", "Software reset", ""] -> [w220] mode=indexing
                      n136 = Enqueue Element(queue=w221, element=w220) -> (queue out=w222:refnum<queue>)  [unwired: 2 in, 2 out]
                    }
                  }
                  frame "Start Task 4" {
                    # ">>Action states Queue Reference >>"
                    # "Action items"
                    n137 = for {
                      shift-right: [w229] -> w224
                      shift-left: w225 -> [w228]
                      tunnel: string[] ["Hardware reset", "Software reset", ""] -> [w227] mode=indexing
                      n138 = Enqueue Element(queue=w228, element=w227) -> (queue out=w229:refnum<queue>)  [unwired: 2 in, 2 out]
                    }
                  }
                  frame "Exit" {
                    # ">>Action states Queue Reference >>"
                    # "Action items"
                    n139 = for {
                      shift-right: [w236] -> w231
                      shift-left: w232 -> [w235]
                      tunnel: string[] ["Hardware reset", "Software reset", "Motor Control", "Pre-Exit", "Exit"] -> [w234] mode=indexing
                      n140 = Enqueue Element(queue=w235, element=w234) -> (queue out=w236:refnum<queue>)  [unwired: 2 in, 2 out]
                    }
                  }
                  frame "Wall follow mode" {
                    # ">>Action states Queue Reference >>"
                    # "Action items"
                    n141 = for {
                      shift-right: [w243] -> w238
                      shift-left: w239 -> [w242]
                      tunnel: string[] ["Hardware reset", "Software reset", ""] -> [w241] mode=indexing
                      n142 = Enqueue Element(queue=w242, element=w241) -> (queue out=w243:refnum<queue>)  [unwired: 2 in, 2 out]
                    }
                  }
                  frame "Camera vision" {
                    # ">>Action states Queue Reference >>"
                    # "Action items"
                    n143 = for {
                      shift-right: [w250] -> w245
                      shift-left: w246 -> [w249]
                      tunnel: string[] ["Hardware reset", "Software reset", "Cam Init", "Cam Acq"] -> [w248] mode=indexing
                      n144 = Enqueue Element(queue=w249, element=w248) -> (queue out=w250:refnum<queue>)  [unwired: 2 in, 2 out]
                    }
                  }
                  frame "Start Drive Straight" {
                    # ">>Action states Queue Reference >>"
                    # "Action items"
                    n145 = for {
                      shift-right: [w257] -> w251
                      shift-left: w253 -> [w256]
                      tunnel: string[] ["Hardware reset", "Software reset", "Forward", ""] -> [w255] mode=indexing
                      n146 = Enqueue Element(queue=w256, element=w255) -> (queue out=w257:refnum<queue>)  [unwired: 2 in, 2 out]
                    }
                  }
                }
              }
              frame "Startup" {
                # ">>State Logic >>"
                n147 = Flush Queue(queue=w258) -> ()  [unwired: 1 in, 3 out]
                n148 = for {
                  shift-right: [w265] -> w260
                  shift-left: w261 -> [w266]
                  tunnel: string[] ["Init", "NavX Calibrate", "Software reset", "Hardware reset", "Motor Control"] -> [w264] mode=indexing
                  n149 = Enqueue Element(queue=w266, element=w264) -> (queue out=w265:refnum<queue>)  [unwired: 2 in, 2 out]
                }
              }
              frame "Task 1" {
                # ">>State Logic >>"
                n150 = Greater Or Equal?(x=w267, y=1.2) -> (x >= y?=w270:bool)
                n151 = Or(x=w272, y=w270) -> (x .or. y?=w273:bool)
                n152 = case shown="False" w273 {
                  tunnel: [string[] ["Forward", "Motor Control", "Ultrasonic read"] string[] ["Software reset", "Hardware reset", "Motor Control"]] -> w276
                  frame False {
                  }
                  frame True {
                  }
                }
                n153 = Flush Queue(queue=w269) -> ()  [unwired: 1 in, 3 out]
                n154 = Select(t=TLB_MHL_States."Idle" ("Enum"), s=w273, f=TLB_MHL_States."Task 1" ("Enum")) -> (s? t:f=w277:T5)
                n155 = for {
                  shift-right: [w283] -> w274
                  shift-left: w275 -> [w284]
                  tunnel: w276 -> [w282] mode=indexing
                  n156 = Enqueue Element(queue=w284, element=w282) -> (queue out=w283:refnum<queue>)  [unwired: 2 in, 2 out]
                }
              }
              frame "Task 2" {
                # ">>State Logic >>"
                n157 = Flush Queue(queue=w286) -> ()  [unwired: 1 in, 3 out]
                n158 = case shown="True" w289 {
                  tunnel: [w296 string[] ["Hardware reset", "Software reset", "Motor control"]] -> w288
                  tunnel: w287 -> [w295 _]
                  frame False {
                    n159 = case shown="False" w295 {
                      tunnel: [string[] ["Stop", "Ultrasonic read", "Motor Control"] string[] ["Reverse", "Ultrasonic read", "Motor control"]] -> w296
                      frame False {
                      }
                      frame True {
                      }
                    }
                  }
                  frame True {
                  }
                }
                n160 = Select(t=TLB_MHL_States."Idle" ("Enum"), s=w289, f=TLB_MHL_States."Task 2" ("Enum")) -> (s? t:f=w292:T5)
                n161 = for {
                  shift-right: [w301] -> w291
                  shift-left: w290 -> [w302]
                  tunnel: w288 -> [w300] mode=indexing
                  n162 = Enqueue Element(queue=w302, element=w300) -> (queue out=w301:refnum<queue>)  [unwired: 2 in, 2 out]
                }
              }
              frame "Task 3" {
                n163 = Less Or Equal?(x=w303, y=-1.15) -> (x <= y?=w307:bool)
                n164 = Flush Queue(queue=w305) -> ()  [unwired: 1 in, 3 out]
                n165 = Or(x=w307, y=w308) -> (x .or. y?=w309:bool)
                n166 = case shown="False" w309 {
                  tunnel: [string[] ["Rotate CW", "Motor Control"] string[] ["Software reset", "Hardware reset", "Motor Control"]] -> w315
                  frame False {
                  }
                  frame True {
                  }
                }
                n167 = for {
                  shift-right: [w317] -> w313
                  shift-left: w314 -> [w318]
                  tunnel: w315 -> [w316] mode=indexing
                  n168 = Enqueue Element(queue=w318, element=w316) -> (queue out=w317:refnum<queue>)  [unwired: 2 in, 2 out]
                }
                n169 = Select(t=TLB_MHL_States."Idle" ("Enum"), s=w309, f=TLB_MHL_States."Task 3" ("Enum")) -> (s? t:f=w310:T5)
              }
              frame "Task 4" {
                n170 = Flush Queue(queue=w321) -> ()  [unwired: 1 in, 3 out]
                n171 = case shown="True" w323 {
                  tunnel: [string[] ["Forward", "Ultrasonic read", "Motor Control"] string[] ["Stop", "Hardware reset", "Software reset", "Motor Control"]] -> w324
                  frame False {
                  }
                  frame True {
                  }
                }
                n172 = for {
                  shift-right: [w333] -> w326
                  shift-left: w325 -> [w334]
                  tunnel: w324 -> [w332] mode=indexing
                  n173 = Enqueue Element(queue=w334, element=w332) -> (queue out=w333:refnum<queue>)  [unwired: 2 in, 2 out]
                }
                n174 = Select(t=TLB_MHL_States."Task 4a" ("Enum"), s=w323, f=TLB_MHL_States."Task 4" ("Enum")) -> (s? t:f=w329:T5)
              }
              frame "Task 4a" {
                n175 = Greater Or Equal?(x=w335, y=0.5) -> (x >= y?=w339:bool)
                n176 = Flush Queue(queue=w336) -> ()  [unwired: 1 in, 3 out]
                n177 = case shown="True" w339 {
                  tunnel: [string[] ["Right", "Motor Control"] string[] ["Stop", "Hardware reset", "Software reset", "Motor Control"]] -> w342
                  frame False {
                  }
                  frame True {
                  }
                }
                n178 = for {
                  shift-right: [w349] -> w340
                  shift-left: w341 -> [w350]
                  tunnel: w342 -> [w348] mode=indexing
                  n179 = Enqueue Element(queue=w350, element=w348) -> (queue out=w349:refnum<queue>)  [unwired: 2 in, 2 out]
                }
                n180 = Select(t=TLB_MHL_States."Task 4b" ("Enum"), s=w339, f=TLB_MHL_States."Task 4a" ("Enum")) -> (s? t:f=w343:T5)
              }
              frame "Task 4b" {
                n181 = Flush Queue(queue=w352) -> ()  [unwired: 1 in, 3 out]
                n182 = Greater Or Equal?(x=w351, y=0.75) -> (x >= y?=w354:bool)
                n183 = case shown="False" w354 {
                  tunnel: [string[] ["Forward", "Motor control"] string[] ["Stop", "Hardware reset", "Software reset"]] -> w359
                  frame False {
                  }
                  frame True {
                  }
                }
                n184 = for {
                  shift-right: [w365] -> w357
                  shift-left: w358 -> [w366]
                  tunnel: w359 -> [w364] mode=indexing
                  n185 = Enqueue Element(queue=w366, element=w364) -> (queue out=w365:refnum<queue>)  [unwired: 2 in, 2 out]
                }
                n186 = Select(t=TLB_MHL_States."Task 4c" ("Enum"), s=w354, f=TLB_MHL_States."Task 4b" ("Enum")) -> (s? t:f=w356:T5)
              }
              frame "Task 4c" {
                n187 = Flush Queue(queue=w368) -> ()  [unwired: 1 in, 3 out]
                n188 = Less Or Equal?(x=w367, y=-0.65) -> (x <= y?=w370:bool)
                n189 = case shown="False" w370 {
                  tunnel: [string[] ["Left", "Motor Control"] string[] ["Stop", "Hardware reset", "Software reset", "Motor Control"]] -> w375
                  frame False {
                  }
                  frame True {
                  }
                }
                n190 = for {
                  shift-right: [w381] -> w372
                  shift-left: w373 -> [w382]
                  tunnel: w375 -> [w380] mode=indexing
                  n191 = Enqueue Element(queue=w382, element=w380) -> (queue out=w381:refnum<queue>)  [unwired: 2 in, 2 out]
                }
                n192 = Select(t=TLB_MHL_States."Task 4d" ("Enum"), s=w370, f=TLB_MHL_States."Task 4c" ("Enum")) -> (s? t:f=w374:T5)
              }
              frame "Task 4d" {
                n193 = Flush Queue(queue=w384) -> ()  [unwired: 1 in, 3 out]
                n194 = Or(x=w387, y=w386) -> (x .or. y?=w385:bool)
                n195 = case shown="True" w385 {
                  tunnel: [string[] ["Forward", "Ultrasonic Read", "Motor Control"] string[] ["Stop", "Hardware reset", "Software reset", "Motor Control"]] -> w391
                  frame False {
                  }
                  frame True {
                  }
                }
                n196 = for {
                  shift-right: [w397] -> w389
                  shift-left: w390 -> [w398]
                  tunnel: w391 -> [w396] mode=indexing
                  n197 = Enqueue Element(queue=w398, element=w396) -> (queue out=w397:refnum<queue>)  [unwired: 2 in, 2 out]
                }
                n198 = Select(t=TLB_MHL_States."Idle" ("Enum"), s=w385, f=TLB_MHL_States."Task 4d" ("Enum")) -> (s? t:f=w388:T5)
              }
              frame "Reset" {
                n199 = for {
                  shift-right: [w405] -> w400
                  shift-left: w401 -> [w406]
                  tunnel: string[] ["Software reset", "Hardware reset", "Motor Control"] -> [w404] mode=indexing
                  n200 = Enqueue Element(queue=w406, element=w404) -> (queue out=w405:refnum<queue>)  [unwired: 2 in, 2 out]
                }
              }
              frame "Wall follow mode" {
                n201 = Flush Queue(queue=w408) -> ()  [unwired: 1 in, 3 out]
                n202 = case shown="False" w409 {
                  tunnel: [string[] ["IR Sensor Read", "Calculate", "Forward", "Motor Control"] string[] ["Hardware reset", "Software reset", "Motor Control"]] -> w410
                  frame False {
                  }
                  frame True {
                  }
                }
                n203 = for {
                  shift-right: [w419] -> w412
                  shift-left: w411 -> [w420]
                  tunnel: w410 -> [w418] mode=indexing
                  n204 = Enqueue Element(queue=w420, element=w418) -> (queue out=w419:refnum<queue>)  [unwired: 2 in, 2 out]
                }
                n205 = Select(t=TLB_MHL_States."Idle" ("Enum"), s=w409, f=TLB_MHL_States."Wall follow mode" ("Enum")) -> (s? t:f=w414:T5)
              }
              frame "Autodrive" {
                # ">>>Return to idle event>>>"
                n206 = Flush Queue(queue=w430) -> ()  [unwired: 1 in, 3 out]
                n207 = Boolean To (0,1)(Boolean=w426) -> (0, 1=w428:i16)
                n208 = Boolean To (0,1)(Boolean=w425) -> (0, 1=w427:i16)
                n209 = formula code="int8  out;\nif (detect == 0 && stop == 0)\nout = 0;\n\nelse if (detect == 1 && stop == 0)\nout = 1;\n\nelse if (detect == 0 && stop == 1)\nout = 2;\n\nelse\nout = 0;"("stop"=w428, "detect"=w427) -> ("out"=w421:i8)
                n210 = case shown="0, Default" w421 {
                  tunnel: [string[] ["Forward", "Ultrasonic read"] string[] ["Hardware reset", "Software reset", "Rotate Clockwise", ""] string[] ["Stop", "Hardware reset", "Software reset", "Motor Control"]] -> w424
                  frame 0, Default {
                  }
                  frame 1 {
                  }
                  frame 2 {
                  }
                }
                n211 = call "FGV DBL.vi"("Init/Read/Write State"=States_for_Action_Engine."Write", "Input node"=w421) -> ()  [unwired: 1 in, 2 out]
                n212 = for {
                  shift-right: [w440] -> w432
                  shift-left: w431 -> [w441]
                  tunnel: w424 -> [w439] mode=indexing
                  n213 = Enqueue Element(queue=w441, element=w439) -> (queue out=w440:refnum<queue>)  [unwired: 2 in, 2 out]
                }
                n214 = case shown="2" w421 {
                  tunnel: [TLB_MHL_States."Autodrive" ("Enum") TLB_MHL_States."Autodrive a" ("Enum") TLB_MHL_States."Idle" ("Enum")] -> w423
                  frame 0, Default {
                  }
                  frame 1 {
                  }
                  frame 2 {
                  }
                }
              }
              frame "Acquire image" {
                n215 = Flush Queue(queue=w443) -> ()  [unwired: 1 in, 3 out]
                n216 = case shown="True" w444 {
                  tunnel: [string[] ["Cam Acq"] string[] ["Hardware reset", "Software reset", "Cam Exit", ""]] -> w448
                  frame False {
                  }
                  frame True {
                  }
                }
                n217 = for {
                  shift-right: [w454] -> w446
                  shift-left: w447 -> [w455]
                  tunnel: w448 -> [w453] mode=indexing
                  n218 = Enqueue Element(queue=w455, element=w453) -> (queue out=w454:refnum<queue>)  [unwired: 2 in, 2 out]
                }
                n219 = Select(t=TLB_MHL_States."Idle" ("Enum"), s=w444, f=TLB_MHL_States."Acquire image" ("Enum")) -> (s? t:f=w445:T5)
              }
              frame "Processing" {
              }
              frame "Shutdown" {
                # ">>State Logic >>"
                n220 = for {
                  shift-right: [w464] -> w459
                  shift-left: w460 -> [w465]
                  tunnel: string[] ["Software reset", "Hardware reset", "Motor Control", "Cam Exit", "Pre-Exit", "Exit"] -> [w463] mode=indexing
                  n221 = Enqueue Element(queue=w465, element=w463) -> (queue out=w464:refnum<queue>)  [unwired: 2 in, 2 out]
                }
              }
              frame "None" {
              }
              frame "Autodrive a" {
                n222 = Greater Or Equal?(x=w468, y=80.0) -> (x >= y?=w470:bool)
                n223 = Or(x=w469, y=w470) -> (x .or. y?=w471:bool)
                n224 = case shown="True" w471 {
                  tunnel: [string[] ["Rotate CW", "Ultrasonic read", ""] string[] ["Stop", "Hardware reset", "Software reset", ""]] -> w479
                  frame False {
                  }
                  frame True {
                  }
                }
                n225 = for {
                  shift-right: [w485] -> w481
                  shift-left: w480 -> [w486]
                  tunnel: w479 -> [w484] mode=indexing
                  n226 = Enqueue Element(queue=w486, element=w484) -> (queue out=w485:refnum<queue>)  [unwired: 2 in, 2 out]
                }
                n227 = Or(x=w469, y=w470) -> (x .or. y?=w472:bool)
                n228 = Select(t=TLB_MHL_States."Idle" ("Enum"), s=w469, f=TLB_MHL_States."Autodrive" ("Enum")) -> (s? t:f=w475:T5)
                n229 = Select(t=w475, s=w472, f=TLB_MHL_States."Autodrive a" ("Enum")) -> (s? t:f=w477:T5)
              }
            }
          }
        }
        n230 = call "FGV DBL.vi"("Init/Read/Write State"=States_for_Action_Engine."Read") -> ("Output"=→"Output":dbl)  [unwired: 2 in, 1 out]
        n231 = local write "GREEN LED State"(w138) -> ()
        "Decision" <- w134
      }
      n232 = while {
        shift-right: [w103] -> _
        shift-left: _ -> [w104]
        shift-right: [w102] -> _
        shift-left: _ -> [w101]
        stop <- w110 stop-if-true
        (unwired) TRUE
        # "LED Blinker Loop"
        n233 = case shown="\"BLINK\"" "GREEN LED State" {
          tunnel: [FALSE TRUE w118] -> w106
          tunnel: w104 -> [_ _ w118]
          tunnel: [_ _ w119] -> w103
          frame "OFF", Default {
          }
          frame "ON" {
          }
          frame "BLINK" {
            n234 = Not(x=w118) -> (.not. x?=w119:bool)
          }
        }
        n235 = case shown="\"OFF\", Default" "RED LED State" {
          tunnel: [FALSE TRUE w114] -> w105
          tunnel: [_ _ w115] -> w102
          tunnel: w101 -> [_ _ w114]
          frame "OFF", Default {
          }
          frame "ON" {
          }
          frame "BLINK" {
            n236 = Not(x=w114) -> (.not. x?=w115:bool)
          }
        }
        n237 = local write "Green LED"(w106) -> ()
        n238 = local write "Red LED"(w105) -> ()
        n239 = call "FGV Bool.vi"("Init/Read/Write State"=States_for_Action_Engine."Read") -> ("Output node"=w110:bool)  [unwired: 2 in, 1 out]
        n240 = Wait (ms)(milliseconds to wait=u32 500) -> ()  [unwired: 1 out]
      }
      n241 = call <vilib>:"DIO Close.vi"("DIO Info In"=w5) -> ()  [unwired: 10 in, 1 out]
      n242 = call <vilib>:"DIO Close.vi"("error in (no error)"=w22, "DIO Info In"=w28) -> ()  [unwired: 9 in, 1 out]
      n243 = call <vilib>:"DIO Close.vi"("error in (no error)"=w20, "DIO Info In"=w24) -> ()  [unwired: 9 in, 1 out]
      n244 = call <vilib>:"DIO Close.vi"("error in (no error)"=w10, "DIO Info In"=w15) -> ()  [unwired: 9 in, 1 out]
      n245 = call <vilib>:"DIO Close.vi"("error in (no error)"=w8, "DIO Info In"=w14) -> ()  [unwired: 9 in, 1 out]
      n246 = Merge Errors "Merge Errors"(w54, w53) -> (w35:errorcluster)
      n247 = Merge Errors(w39, w35) -> (w30:errorcluster)
      n248 = Destroy User Event(user event=w57, error in=w30) -> ()  [unwired: 1 out]
      n249 = Destroy User Event(user event=w58, error in=w30) -> ()  [unwired: 1 out]
      n250 = Unregister For Events(event registration refnum=w49, error in=w30) -> ()  [unwired: 1 out]
      n251 = Release Queue(queue=w32, error in (no error)=w30) -> (error out=→"error out":errorcluster)  [unwired: 1 in, 2 out]
      n252 = call <vilib>:"NavX Close.vi"("NavX Info In"=w4) -> ()  [unwired: 10 in, 1 out]
      n253 = Release Queue(queue=w48, error in (no error)=w30) -> ()  [unwired: 1 in, 3 out]
    }
    frame #2 {
      (unwired) T15."INIT" ("States")
      n254 = call "New motor Control integrated remodeled state based.vi"() -> ()  [unwired: 3 in, 2 out]
    }
    frame #3 {
    }
  }
